vi "流程写入.vi"(11 "添加的路径":path) -> ()   [LabVIEW 2016, in "斯坦道CODMn新电路板.lvlib"]
uses:
  <vilib>/Utility/miscctls.llb/LVPointTypeDef.ctl
panel:
  in  "加标回收":bool
  in  "平行样":bool
  in  "关闭":bool
  out "字符串":string
  in  "跨度核查":bool
  in  "标样核查":bool
  in  "空白测试":bool
  in  "零点核查":bool
  in  "水样测量":bool=TRUE
  in  "写入":bool
  in  "参数下拉列表":u16(ring)=21 items=["总磷"=0, "总氮"=1, "CODMn"=21]
  in  "量程下拉列表":enum16{"低量程", "高量程"}(ring)
  # "请选择要写入的流程"
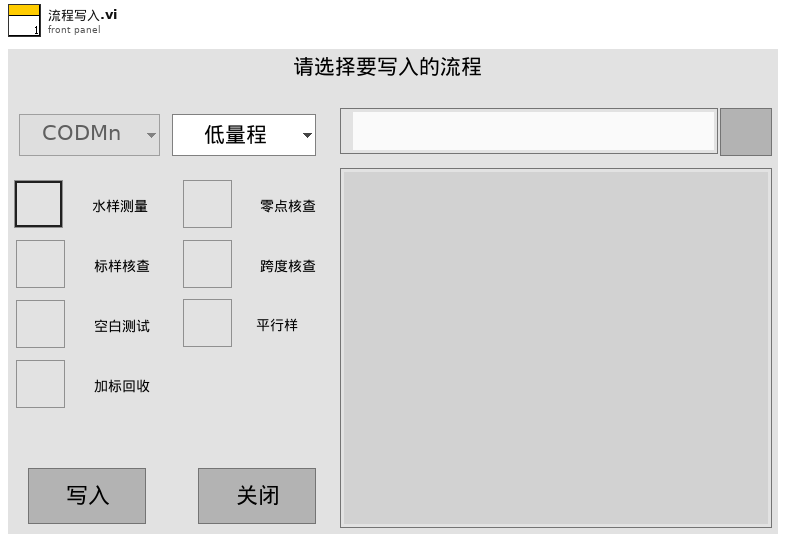
[diagram p1: front panel]
types:
  T1 = typedef "LVPointTypeDef.ctl" = cluster{"Horizontal":i16, "Vertical":i16}
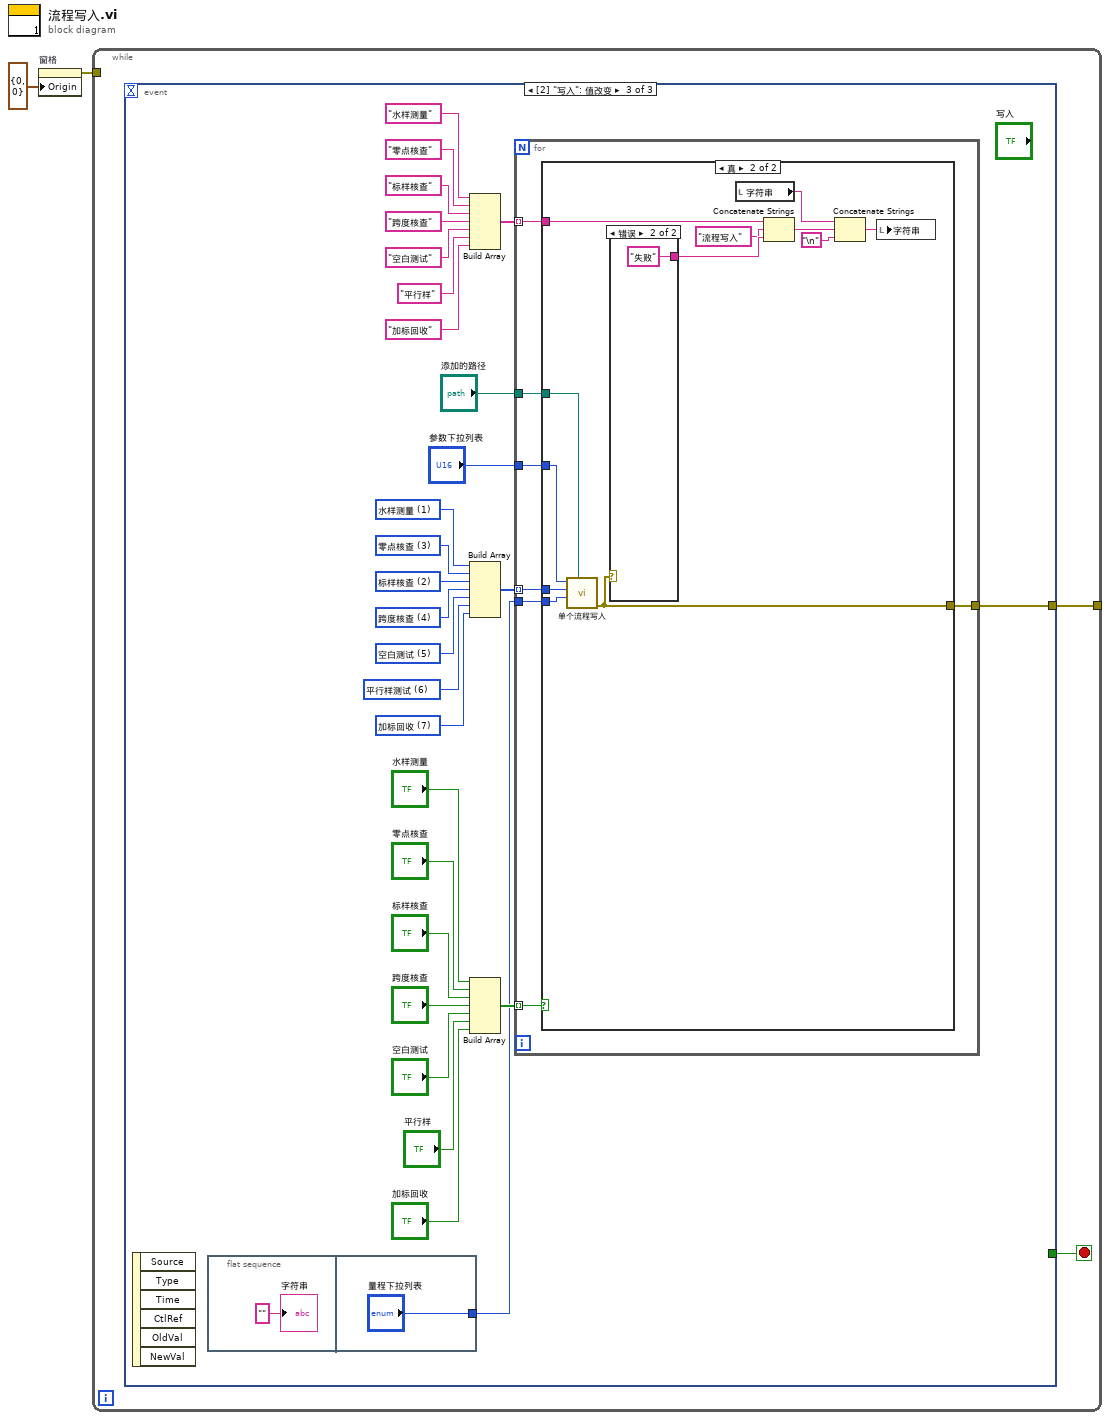
[diagram p0: block diagram]
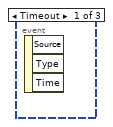
[diagram p2: hidden frame]
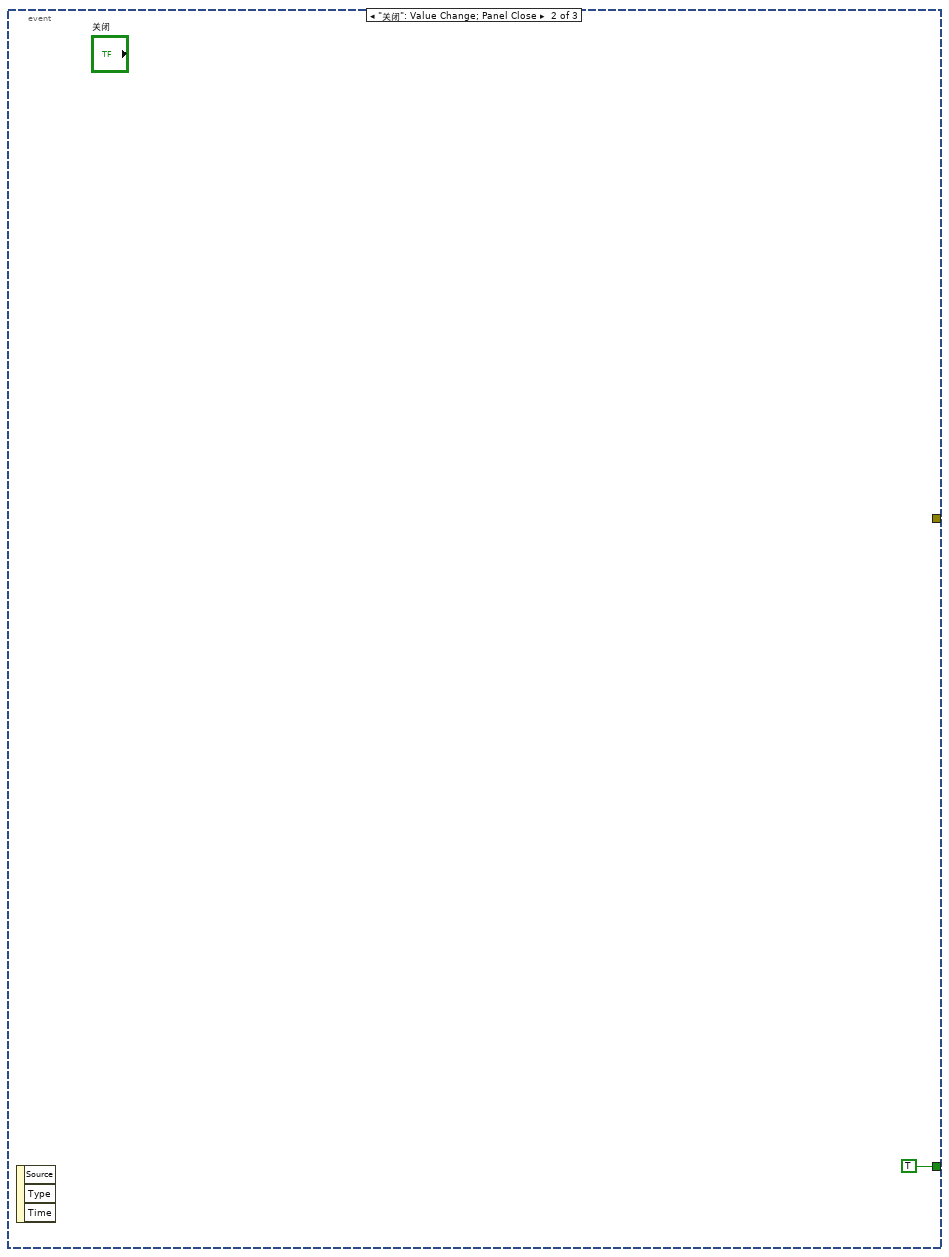
[diagram p3: hidden frame]
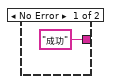
[diagram p5: hidden frame]
diagram:
  n1 = property on="窗格" class="Pane"("Origin"=T1 {"Horizontal"=0, "Vertical"=0} ("原点")) -> (error out=w1:errorcluster)  [unwired: 2 in, 1 out]
  n2 = while {
    tunnel: w1 -> [_]
    tunnel: [w3] -> _
    stop <- w4 stop-if-true
    n3 = event shown="[2] \"写入\": 值改变" {
      selector: _ -> [_ _ _]
      dyn-events: _ -> [_ _ _]
      timeout: _ -> [_ _ _]
      tunnel: [_ TRUE _] -> w4
      tunnel: [_ _ w6] -> w3
      event Timeout {
        n4 = event-data() -> ()  [unwired: 1 in, 3 out]
      }
      event "关闭": Value Change; Panel Close {
        n5 = event-data() -> ()  [unwired: 1 in, 3 out]
      }
      event "写入": Value Change {
        w24 = u16 7 items=["", "水样测量", "标样核查", "零点核查", "跨度核查", "空白测试", "平行样测试", "加标回收", "校零", "校标"] ("测量模式")
        w23 = u16 6 items=["", "水样测量", "标样核查", "零点核查", "跨度核查", "空白测试", "平行样测试", "加标回收", "校零", "校标"] ("测量模式")
        w22 = u16 5 items=["", "水样测量", "标样核查", "零点核查", "跨度核查", "空白测试", "平行样测试", "加标回收", "校零", "校标"] ("测量模式")
        w21 = u16 4 items=["", "水样测量", "标样核查", "零点核查", "跨度核查", "空白测试", "平行样测试", "加标回收", "校零", "校标"] ("测量模式")
        w20 = u16 2 items=["", "水样测量", "标样核查", "零点核查", "跨度核查", "空白测试", "平行样测试", "加标回收", "校零", "校标"] ("测量模式")
        w19 = u16 3 items=["", "水样测量", "标样核查", "零点核查", "跨度核查", "空白测试", "平行样测试", "加标回收", "校零", "校标"] ("测量模式")
        w18 = u16 1 items=["", "水样测量", "标样核查", "零点核查", "跨度核查", "空白测试", "平行样测试", "加标回收", "校零", "校标"] ("测量模式")
        n6 = event-data() -> ()  [unwired: 1 in, 6 out]
        n7 = flat-sequence {
          tunnel: ["量程下拉列表"] -> w7
          frame #0 {
            "字符串" <- ""
          }
          frame #1 {
          }
        }
        n8 = Build Array("水样测量", "零点核查", "标样核查", "跨度核查", "空白测试", "平行样", "加标回收") -> (w33:string[])
        n9 = Build Array(w18, w19, w20, w21, w22, w23, w24) -> (w32:u16[])
        n10 = Build Array("水样测量", "零点核查", "标样核查", "跨度核查", "空白测试", "平行样", "加标回收") -> (w17:bool[])
        n11 = for {
          tunnel: w17 -> [w40] mode=indexing
          tunnel: w32 -> [w38] mode=indexing
          tunnel: w33 -> [w39] mode=indexing
          tunnel: "添加的路径" -> [w37]
          tunnel: "参数下拉列表" -> [w36]
          tunnel: w7 -> [w35]
          tunnel: [w34] -> w6
          n12 = case shown="真" w40 {
            tunnel: w39 -> [_ w46]
            tunnel: w38 -> [_ w45]
            tunnel: w37 -> [_ w44]
            tunnel: w36 -> [_ w43]
            tunnel: w35 -> [_ w42]
            tunnel: [_ w41] -> w34
            frame False {
            }
            frame True {
              n13 = call "单个流程写入.vi"("添加的路径"=w44, "量程"=w42, "测量模式"=w45, "测量参数"=w43) -> ("error out"=w41:errorcluster)  [unwired: 6 in, 1 out]
              n14 = case shown="错误" w41 {
                tunnel: ["成功" "失败"] -> w49
                frame No Error {
                }
                frame Error {
                }
              }
              n15 = local read "字符串"() -> (w47:string)
              n16 = Concatenate Strings(w46, "流程写入", w49) -> (w50:string)
              n17 = Concatenate Strings(w47, w50, "\n") -> (w52:string)
              n18 = local write "字符串"(w52) -> ()
            }
          }
        }
      }
    }
  }
